vi "TIFF_CloseMeta.vi"(8 "error in (no error)":errorcluster, 11 "Input cluster":T1) -> (0 "error out":errorcluster)   [LabVIEW 2025]
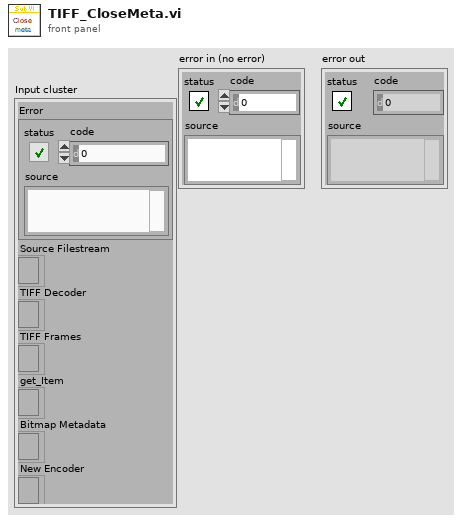
[diagram p1: front panel]
types:
  T1 = cluster{"Error":errorcluster, "Source Filestream":refnum<k24>, "TIFF Decoder":refnum<k24>, "TIFF Frames":refnum<k24>, "get_Item":refnum<k24>, "Bitmap Metadata":refnum<k24>, "New Encoder":refnum<k24>}
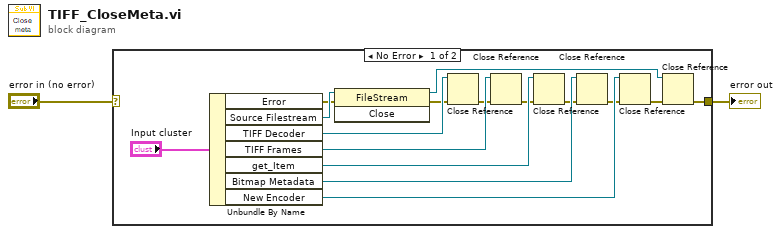
[diagram p0: block diagram]
diagram:
  n1 = case shown="No Error" "error in (no error)" {
    selector: "error in (no error)" -> [_ w19]
    tunnel: [w3 w19] -> w2
    frame No Error {
      n2 = Unbundle By Name("Input cluster") -> ("Error"=w10:errorcluster, "Source Filestream"=w12:refnum<k24>, "TIFF Decoder"=w17:refnum<k24>, "TIFF Frames"=w16:refnum<k24>, "get_Item"=w15:refnum<k24>, "Bitmap Metadata"=w14:refnum<k24>, "New Encoder"=w13:refnum<k24>)
      n3 = invoke class="FileStream" method="Close"(reference=w12, error in=w10) -> (reference out=w11:refnum<k24>, error out=w9:errorcluster)  [unwired: 1 in, 1 out]
      n4 = Close Reference(reference=w17, error in (no error)=w9) -> (error out=w8:errorcluster)
      n5 = Close Reference(reference=w16, error in (no error)=w8) -> (error out=w7:errorcluster)
      n6 = Close Reference(reference=w15, error in (no error)=w7) -> (error out=w6:errorcluster)
      n7 = Close Reference(reference=w14, error in (no error)=w6) -> (error out=w5:errorcluster)
      n8 = Close Reference(reference=w13, error in (no error)=w5) -> (error out=w4:errorcluster)
      n9 = Close Reference(reference=w11, error in (no error)=w4) -> (error out=w3:errorcluster)
    }
    frame Error {
    }
  }
  "error out" <- w2
